vi "v1h_get_NC_dimarray.vi"(3 "error out":errorcluster caption="error in", 5 "refnum in":refnum<file>) -> (0 "error out":errorcluster, 1 "NC_dimarray":cluster{"name":string, "size":u64}[](array[cluster]), 2 "refnum out":refnum<file>)   [LabVIEW 2016]
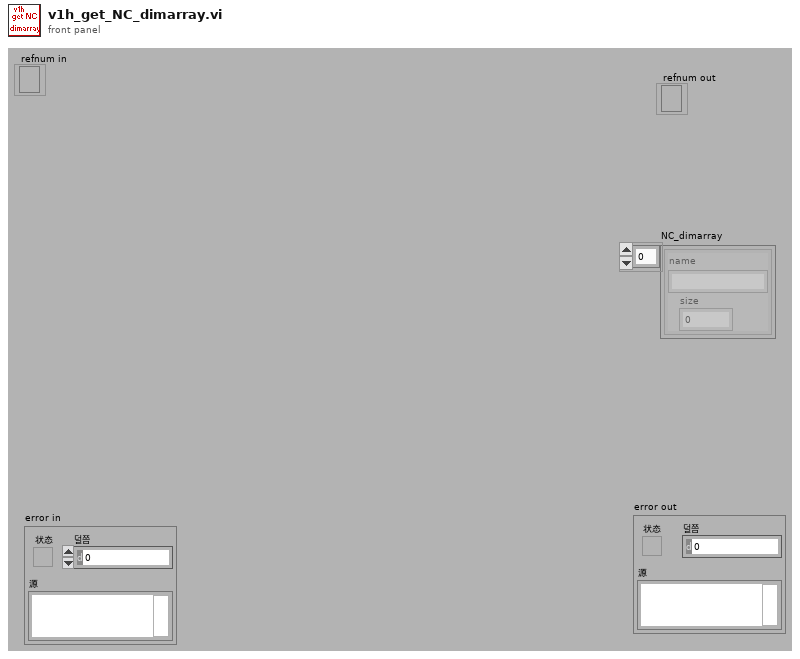
[diagram p1: front panel]
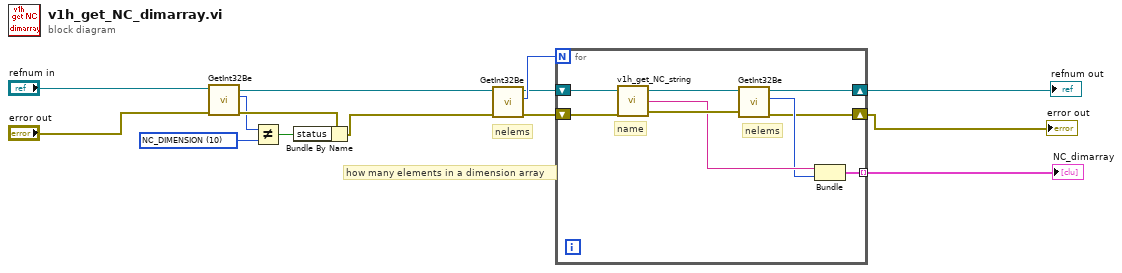
[diagram p0: block diagram]
diagram:
  w6 = u16 10 items=["NC_UNSPECIFIED"=0, "NC_BITFIELD"=7, "NC_STRING"=8, "NC_DIMENSION"=10, "NC_VARIABLE"=11, "NC_ATTRIBUTE"=12] ("NCtype")
  # "how many elements in a dimension array"
  # "nelems"
  n1 = call "GetInt32Be.vi"("error in (no error)"="error out", "refnum in"="refnum in") -> ("error out"=w8:errorcluster, "int32"=w5:i32, "refnum out"=w10:refnum<file>)  [unwired: 3 out]
  n2 = Not Equal?(x=w5, y=w6) -> (x != y?=w9:bool)
  n3 = Bundle By Name(cluster=w8, "status"=w9) -> (w11:errorcluster)
  n4 = call "GetInt32Be.vi"("error in (no error)"=w11, "refnum in"=w10) -> ("error out"=w3:errorcluster, "int32"=w13:i32, "refnum out"=w12:refnum<file>)  [unwired: 3 out]
  n5 = for {
    N: w13 -> [_]
    shift-right: [w20] -> w14
    shift-left: w12 -> [w23]
    tunnel: [w17] -> w1 mode=indexing
    shift-right: [w15] -> w2
    shift-left: w3 -> [w16]
    # "nelems"
    # "name"
    n6 = call "v1h_get_NC_string.vi"("error in (no error)"=w16, "refnum in"=w23) -> ("error out"=w21:errorcluster, "NC_string"=w19:string, "refnum out"=w22:refnum<file>)  [unwired: 1 out]
    n7 = call "GetInt32Be.vi"("error in (no error)"=w21, "refnum in"=w22) -> ("error out"=w15:errorcluster, "int32"=w18:i32, "refnum out"=w20:refnum<file>)  [unwired: 3 out]
    n8 = Bundle("NC_string"=w19, "int32"=w18) -> (w17:cluster{"NC_string":string, "int32":i32})  [unwired: 1 out]
  }
  "refnum out" <- w14
  "error out" <- w2
  "NC_dimarray" <- w1
